vi "UltraStraightDrive.vi"() -> ()   [LabVIEW 2015]
uses:
  Sprocket/src/Refname/Actuators.ctl
  Sprocket/src/Action/Action Name.ctl
  Sprocket/src/Refname/Refname to String (Actuator).vi
  <vilib>/Rock Robotics/WPI/Ultrasonic/WPI_SonarMB1010DigitalRefNum Registry Get.vi
  Main/Robot Global Data.vi
  <vilib>/Rock Robotics/WPI/Ultrasonic/WPI_SonarMB1010DigitalGetRange.vi
  <vilib>/addons/control/pid/pid.llb/PID (DBL).vi
  <vilib>/addons/control/pid/NI_PID_pid.lvlib
  Sprocket/lib/Sprocket.lvlib
panel:
  in  "output range True":cluster{"output high":dbl, "output low":dbl}={"output high"=1.0, "output low"=0.0}
  in  "PID gains True":T1={"proportional gain (Kc)"=0.2, "integral time (Ti, min)"=0.0, "derivative time (Td, min)"=0.0}
  in  "output range False":cluster{"output high":dbl, "output low":dbl}={"output high"=1.0, "output low"=0.0}
  in  "PID gains False":T1={"proportional gain (Kc)"=0.2, "integral time (Ti, min)"=0.0, "derivative time (Td, min)"=0.0}
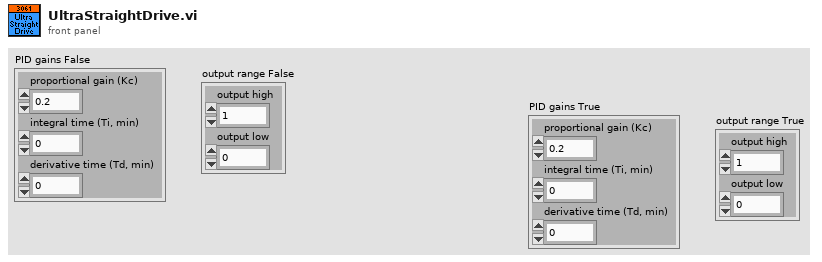
[diagram p1: front panel]
types:
  T1 = cluster{"proportional gain (Kc)":dbl, "integral time (Ti, min)":dbl, "derivative time (Td, min)":dbl}
  T2 = typedef "Sprocket.lvlib/Actuators.ctl" = enum16{"Drive Motors L.Top", "Drive Motors R.Top", "Drive Motors L.Bot", "Drive Motors R.Bot", "Collector Motor", "Collector Solenoid", "Compressor", "SonicShifter", "Gyro", "UltraSonic Front Left", "UltraSonic Back Left"}
  T3 = typedef "WPI_SonarMB1010DigitalDeviceRef.ctl" = cluster{"CounterDevRef":T4, "Scaling factor (s/in)":dbl}
  T4 = typedef "WPI_CounterDevRef.ctl" = cluster{"DevStatus":errorcluster, "CntIndex":T5}
  T5 = typedef "FPGA_CounterCtrSystemIndex.ctl" = enum8{"Ctr 0", "Ctr 1", "Ctr 2", "Ctr 3", "Ctr 4", "Ctr 5", "Ctr 6", "Ctr 7", "Invalid"}
  T6 = typedef "Sprocket.lvlib/Action Name.ctl" = enum16{"No Action", "Drive Train Left", "Drive Train Right", "Drive Train Both", "Collector Motor Eject", "Collector Motor Collect", "Collector Motor Stop", "Collector Extend", "Collector Retract", "Shifter High", "Shifter Low"}
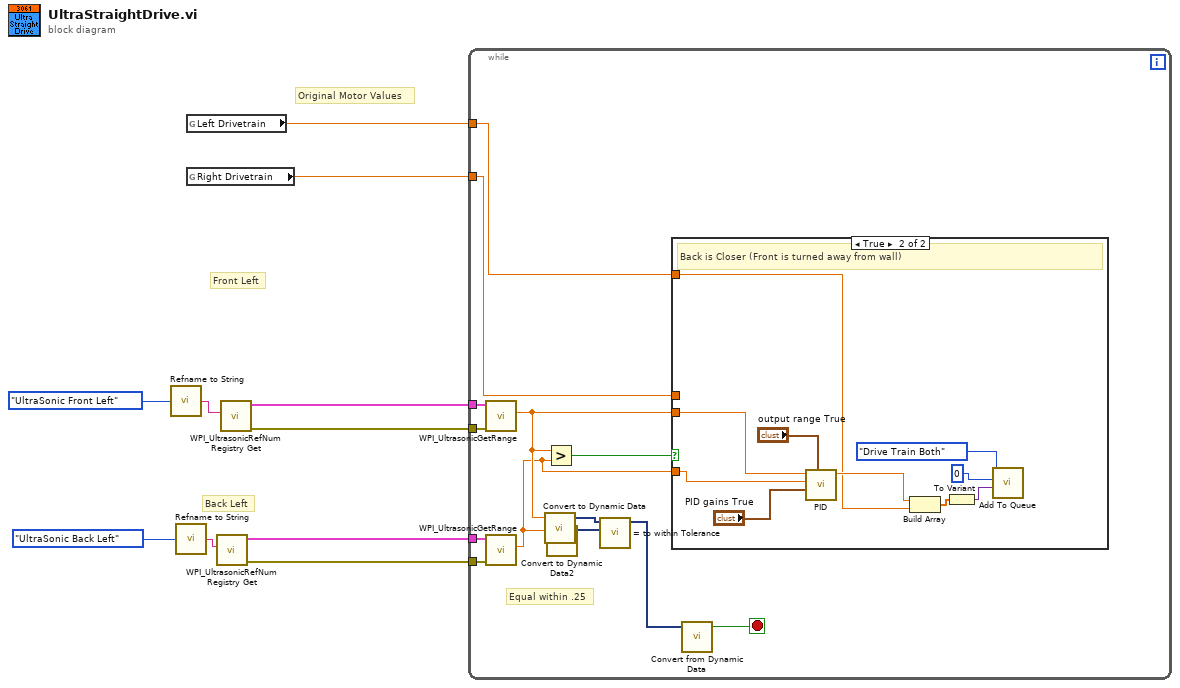
[diagram p0: block diagram]
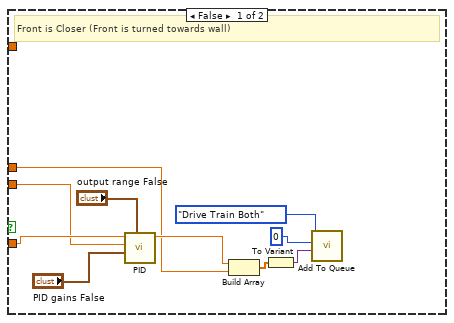
[diagram p2: hidden frame]
diagram:
  # "Original Motor Values"
  # "Back Left"
  # "Front Left"
  n1 = call-poly "Refname to String.vi"("Actuator Refname"=Actuators."UltraSonic Front Left") -> ("Refnum Name"=w4:string)
  n2 = call-poly "Refname to String.vi"("Actuator Refname"=Actuators."UltraSonic Back Left") -> ("Refnum Name"=w3:string)
  n3 = global read "Robot Global Data.vi" "Left Drivetrain"() -> (w6:dbl)
  n4 = global read "Robot Global Data.vi" "Right Drivetrain"() -> (w5:dbl)
  n5 = call-poly <vilib>:"WPI_UltrasonicRefNum Registry Get.vi"("refnum name"=w3) -> ("error out"=w7:errorcluster, "SonarMB1010DigitalDevRef"=w8:T3)  [unwired: 9 in]
  n6 = call-poly <vilib>:"WPI_UltrasonicRefNum Registry Get.vi"("refnum name"=w4) -> ("error out"=w9:errorcluster, "SonarMB1010DigitalDevRef"=w10:T3)  [unwired: 9 in]
  n7 = while {
    tunnel: w10 -> [w23]
    tunnel: w9 -> [w22]
    tunnel: w8 -> [w21]
    tunnel: w7 -> [w20]
    tunnel: w6 -> [w17]
    tunnel: w5 -> [w18]
    stop <- w15 stop-if-true
    # "Equal within .25"
    n8 = call-poly <vilib>:"WPI_UltrasonicGetRange.vi"("error in"=w22, "SonarMB1010DigitalDevRef"=w23) -> ("Distance"=w12:dbl)  [unwired: 7 in, 2 out]
    n9 = call-poly <vilib>:"WPI_UltrasonicGetRange.vi"("error in"=w20, "SonarMB1010DigitalDevRef"=w21) -> ("Distance"=w11:dbl)  [unwired: 7 in, 2 out]
    n10 = call "Convert to Dynamic Data"("Double"=w12) -> ("Dynamic Data Type"=w13:dynamicdata)  [unwired: 3 in]
    n11 = Greater?(x=w12, y=w11) -> (0:w19:bool)
    n12 = call "Convert to Dynamic Data2"("Double"=w11) -> ("Dynamic Data Type"=w14:dynamicdata)  [unwired: 3 in]
    n13 = call "= to within Tolerance"("Operand 2"=w14, "Operand 1"=w13) -> ("Result"=w16:dynamicdata)  [unwired: 8 in, 1 out]
    n14 = case shown="True" w19 {
      tunnel: w11 -> [w32 w36]
      tunnel: w12 -> [w31 w35]
      tunnel: w18 -> [w24 _]
      tunnel: w17 -> [_ w34]
      frame False {
        # "Front is Closer (Front is turned towards wall)"
        n15 = call-poly <vilib>:"PID.vi"("output range"="output range False", "PID gains"="PID gains False", "process variable"=w31, "setpoint"=w32) -> ("output"=w25:dbl)  [unwired: 6 in, 1 out]
        n16 = Build Array(w25, w24) -> (w26:dbl[])
        n17 = To Variant(anything=w26) -> (Variant=w27:variant)
        n18 = call "Add To Queue.vi"("Data"=w27, "Priority"=0, "Action"=Action_Name."Drive Train Both") -> ()  [unwired: 8 in, 1 out]
      }
      frame True {
        # "Back is Closer (Front is turned away from wall)"
        n19 = call-poly <vilib>:"PID.vi"("output range"="output range True", "PID gains"="PID gains True", "process variable"=w36, "setpoint"=w35) -> ("output"=w37:dbl)  [unwired: 6 in, 1 out]
        n20 = Build Array(w37, w34) -> (w38:dbl[])
        n21 = To Variant(anything=w38) -> (Variant=w39:variant)
        n22 = call "Add To Queue.vi"("Data"=w39, "Priority"=0, "Action"=Action_Name."Drive Train Both") -> ()  [unwired: 8 in, 1 out]
      }
    }
    n23 = call "Convert from Dynamic Data"("Dynamic Data Type"=w16) -> ("Scalar"=w15:bool)  [unwired: 3 in]
  }
